vi "SystemLink_Write.vi"(8 "String":string, 9 "Numeric":dbl, 10 "Boolean":bool, 11 "SL_XControl":T1(xcontrol)) -> ()   [LabVIEW 2019]
uses:
  SL_Subs/SL_XControl.xctl
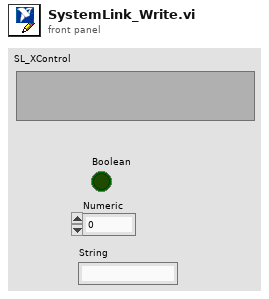
[diagram p1: front panel]
types:
  T1 = cluster{"Tag":string, "Type":string, "Data":string}
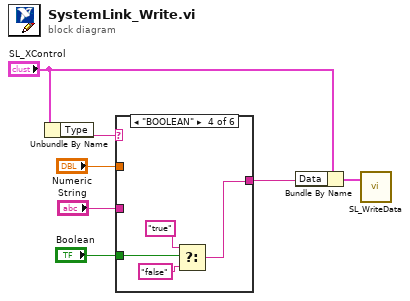
[diagram p0: block diagram]
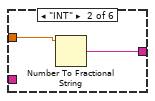
[diagram p3: hidden frame]
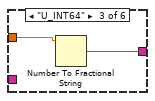
[diagram p4: hidden frame]
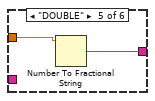
[diagram p5: hidden frame]
diagram:
  n1 = Unbundle By Name("SL_XControl") -> ("Type"=w6:string)
  n2 = case shown="\"BOOLEAN\"" w6 {
    tunnel: "Numeric" -> [_ w10 w12 _ w18 _]
    tunnel: [w8 w9 w11 w13 w17 w19] -> w5
    tunnel: "String" -> [w8 _ _ _ _ w19]
    tunnel: "Boolean" -> [_ _ _ w16 _ _]
    frame Default {
    }
    frame "INT" {
      n3 = Number To Fractional String(number=w10) -> (F-format string=w9:string)  [unwired: 3 in]
    }
    frame "U_INT64" {
      n4 = Number To Fractional String(number=w12) -> (F-format string=w11:string)  [unwired: 3 in]
    }
    frame "BOOLEAN" {
      n5 = Select(t="true", s=w16, f="false") -> (s? t:f=w13:string)
    }
    frame "DOUBLE" {
      n6 = Number To Fractional String(number=w18) -> (F-format string=w17:string)  [unwired: 3 in]
    }
    frame "DATE_TIME" {
      # "Not supported"
    }
  }
  n7 = Bundle By Name(cluster="SL_XControl", "Data"=w5) -> (w2:T1)
  n8 = call "SL_WriteData.vi"("Tag"=w2) -> ()  [unwired: 11 in]
